vi "Measure aggregator.vi"(8 "error in (no error)":errorcluster, 9 "Card #":u8, 11 "VISA resource name":refnum<visa-resource-name>) -> (0 "error out":errorcluster, 2 "appended array":sgl[](array[numeric]))   [LabVIEW 2012, in "Universal Power Meter.lvlib" / "Yokogawa WT2X0.lvlib" / "Yokogawa WT2X0.lvclass"]
uses:
  Yokogawa WT2X0.lvclass
  <instrlib>/Yokogawa WT200 Series/Yokogawa WT200 Series.lvlib
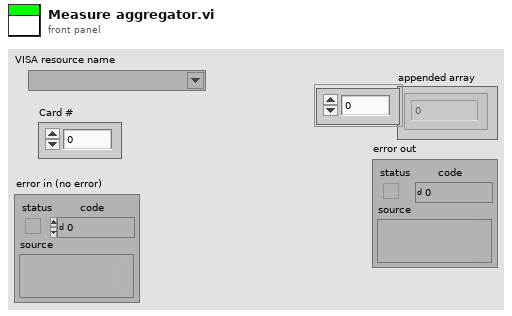
[diagram p1: front panel]
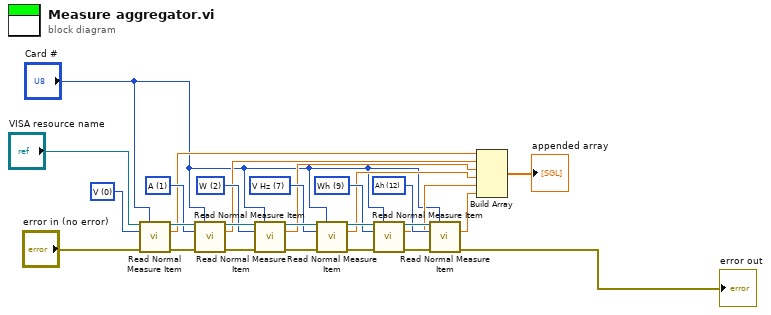
[diagram p0: block diagram]
diagram:
  w17 = u16 12 items=["V", "A", "W", "VA", "var", "PF", "deg", "V Hz", "A Hz", "Wh", "Wh+", "Wh-", "Ah", "Ah+", "Ah-", "Vpk", "Apk", "Math"] ("Measure Item (0: V)")
  w18 = u16 9 items=["V", "A", "W", "VA", "var", "PF", "deg", "V Hz", "A Hz", "Wh", "Wh+", "Wh-", "Ah", "Ah+", "Ah-", "Vpk", "Apk", "Math"] ("Measure Item (0: V)")
  w19 = u16 7 items=["V", "A", "W", "VA", "var", "PF", "deg", "V Hz", "A Hz", "Wh", "Wh+", "Wh-", "Ah", "Ah+", "Ah-", "Vpk", "Apk", "Math"] ("Measure Item (0: V)")
  w20 = u16 2 items=["V", "A", "W", "VA", "var", "PF", "deg", "V Hz", "A Hz", "Wh", "Wh+", "Wh-", "Ah", "Ah+", "Ah-", "Vpk", "Apk", "Math"] ("Measure Item (0: V)")
  w21 = u16 1 items=["V", "A", "W", "VA", "var", "PF", "deg", "V Hz", "A Hz", "Wh", "Wh+", "Wh-", "Ah", "Ah+", "Ah-", "Vpk", "Apk", "Math"] ("Measure Item (0: V)")
  w22 = u16 0 items=["V", "A", "W", "VA", "var", "PF", "deg", "V Hz", "A Hz", "Wh", "Wh+", "Wh-", "Ah", "Ah+", "Ah-", "Vpk", "Apk", "Math"] ("Measure Item (0: V)")
  n1 = call <instrlib>:"Read Normal Measure Item.vi"("VISA resource name"="VISA resource name", "Element (1: Element 1)"="Card #", "Measure Item (0: V)"=w22, "error in (no error)"="error in (no error)") -> ("VISA resource name out"=w27:refnum<visa-resource-name>, "Measure Value"=w9:sgl, "error out"=w16:errorcluster)  [unwired: 8 in, 1 out]
  n2 = call <instrlib>:"Read Normal Measure Item.vi"("VISA resource name"=w27, "Element (1: Element 1)"="Card #", "Measure Item (0: V)"=w21, "error in (no error)"=w16) -> ("VISA resource name out"=w26:refnum<visa-resource-name>, "Measure Value"=w8:sgl, "error out"=w15:errorcluster)  [unwired: 8 in, 1 out]
  n3 = call <instrlib>:"Read Normal Measure Item.vi"("VISA resource name"=w26, "Element (1: Element 1)"="Card #", "Measure Item (0: V)"=w20, "error in (no error)"=w15) -> ("VISA resource name out"=w25:refnum<visa-resource-name>, "Measure Value"=w7:sgl, "error out"=w14:errorcluster)  [unwired: 8 in, 1 out]
  n4 = call <instrlib>:"Read Normal Measure Item.vi"("VISA resource name"=w25, "Element (1: Element 1)"="Card #", "Measure Item (0: V)"=w19, "error in (no error)"=w14) -> ("VISA resource name out"=w24:refnum<visa-resource-name>, "Measure Value"=w6:sgl, "error out"=w13:errorcluster)  [unwired: 8 in, 1 out]
  n5 = call <instrlib>:"Read Normal Measure Item.vi"("VISA resource name"=w24, "Element (1: Element 1)"="Card #", "Measure Item (0: V)"=w18, "error in (no error)"=w13) -> ("VISA resource name out"=w23:refnum<visa-resource-name>, "Measure Value"=w5:sgl, "error out"=w12:errorcluster)  [unwired: 8 in, 1 out]
  n6 = call <instrlib>:"Read Normal Measure Item.vi"("VISA resource name"=w23, "Element (1: Element 1)"="Card #", "Measure Item (0: V)"=w17, "error in (no error)"=w12) -> ("Measure Value"=w4:sgl, "error out"=→"error out":errorcluster)  [unwired: 8 in, 2 out]
  n7 = Build Array(w9, w8, w7, w6, w5, w4) -> (→"appended array":sgl[])
